vi "Get All Keys and Values.vi"(8 "error in":errorcluster, 11 "Cluster In":variant) -> (0 "error out":errorcluster, 1 "values":variant[](array[variant]), 2 "keys":string[](array[string]), 3 "Cluster Out":variant)   [LabVIEW 2017, in "Cluster Manipulation API.lvlib"]
doc: "Returns an array of all of the keys and an array of their corresponding values. Elements are correlated by index, so the key at a given index corresponds to the value at the same index."
uses:
  Cluster Manipulation API.lvlib
  <vilib>/Utility/Data Type/NI_Data Type.lvlib
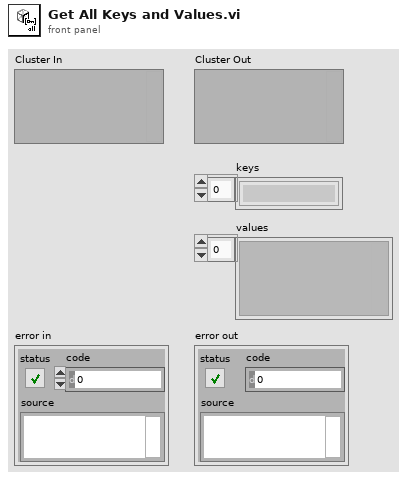
[diagram p1: front panel]
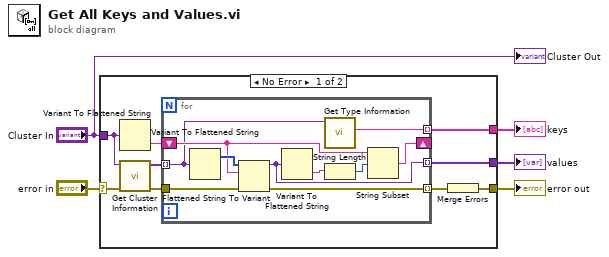
[diagram p0: block diagram]
diagram:
  n1 = case shown="No Error" "error in" {
    selector: "error in" -> [w9 w25]
    tunnel: "Cluster In" -> [w10 _]
    tunnel: [w8 w25] -> w3
    tunnel: [w7 _] -> w2
    tunnel: [w6 _] -> w1
    frame No Error {
      n2 = Variant To Flattened String(Variant=w10) -> (data string=w11:string)  [unwired: 1 out]
      n3 = call <vilib>:"Get Cluster Information.vi"("error in (no error)"=w9, "Variant"=w10) -> ("error out"=w13:errorcluster, "Cluster Elements"=w12:variant[])  [unwired: 8 in]
      n4 = for {
        tunnel: w12 -> [w16] mode=indexing
        tunnel: [w23] -> w7 mode=indexing
        shift-right: [w19] -> _
        shift-left: w11 -> [w22]
        tunnel: w13 -> [w18]
        tunnel: [w17] -> w14 mode=indexing
        tunnel: [w15] -> w6 mode=indexing
        n5 = Variant To Flattened String(Variant=w16) -> (1:w24:i16[])  [unwired: 1 out]
        n6 = Flattened String To Variant(4:w18, 6:w22, 7:w24) -> (0:w17:errorcluster, 3:w23:variant)
        n7 = Variant To Flattened String(Variant=w23) -> (data string=w21:string)  [unwired: 1 out]
        n8 = call <vilib>:"Get Type Information.vi"("Variant"=w16) -> ("Name"=w15:string)  [unwired: 6 in, 4 out]
        n9 = String Length(string=w21) -> (length=w20:i32)
        n10 = String Subset(string=w22, offset (0)=w20) -> (substring=w19:string)  [unwired: 1 in]
      }
      n11 = Merge Errors(w14) -> (w8:errorcluster)
    }
    frame Error {
    }
  }
  "keys" <- w1
  "values" <- w2
  "error out" <- w3
  "Cluster Out" <- "Cluster In"
